vi "Lab_1_Mione_1.vi"() -> ()   [LabVIEW 2018]
panel:
  in  "Current":string
  in  "Temperature":string
  in  "Comment":string
  in  "file path (use dialog)":path
  out "acquiring":bool
  in  "stop acquisition":bool
  in  "Resolution":string(combo)
  in  "Averages":string(combo)
  in  "Enum":T1(ring)=enum."command"
  in  "enter":bool
  in  "stop":bool
  in  "Stop [nm]":dbl
  out "Stop [THz]":dbl
  out "Start [THz]":dbl
  in  "Start [nm]":dbl
  in  "8000/8002":bool
  out "read buffer":string
  in  "Check instruction":string
  out "Initialized":bool
  out "ID number":string
  out "XY Graph":cluster{dbl[], dbl[]}(graph)
  # "Acquisition parameters"
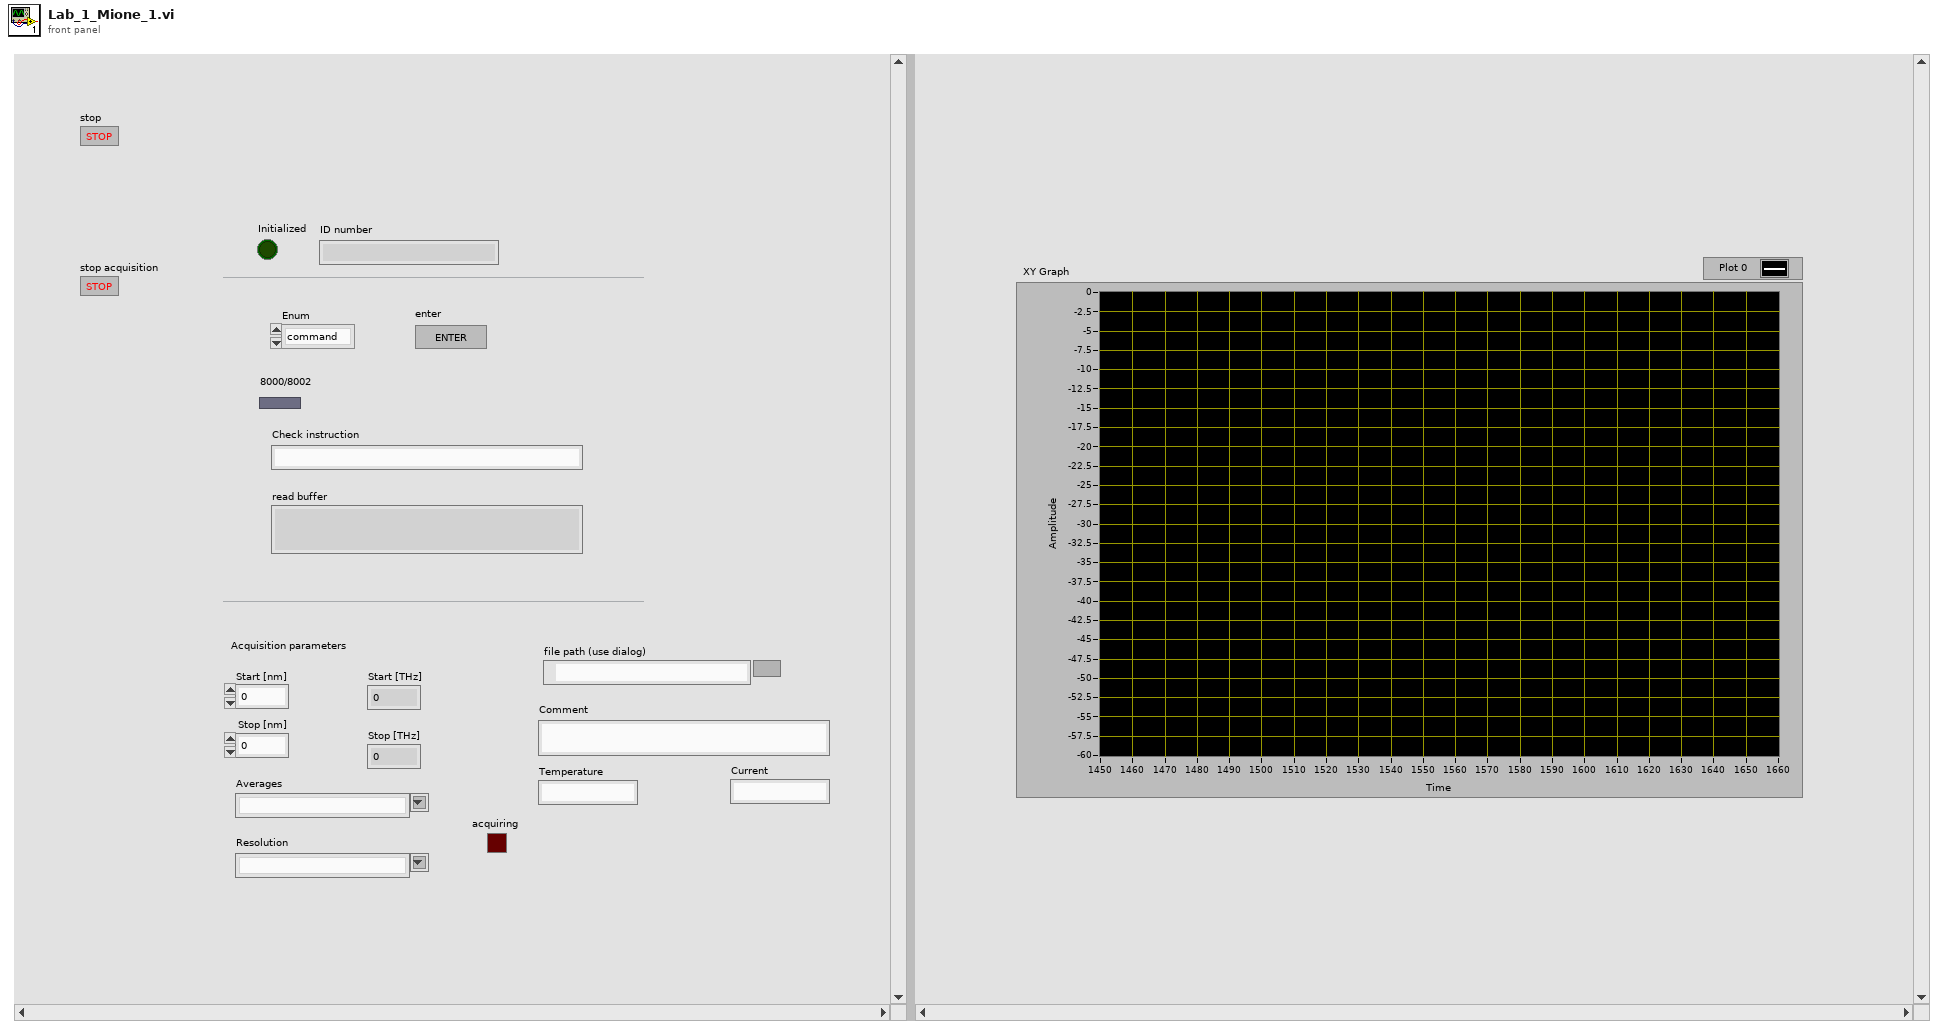
[diagram p1: front panel]
types:
  T1 = enum16{"acquire", "wait", "command", "query", "initialize"}
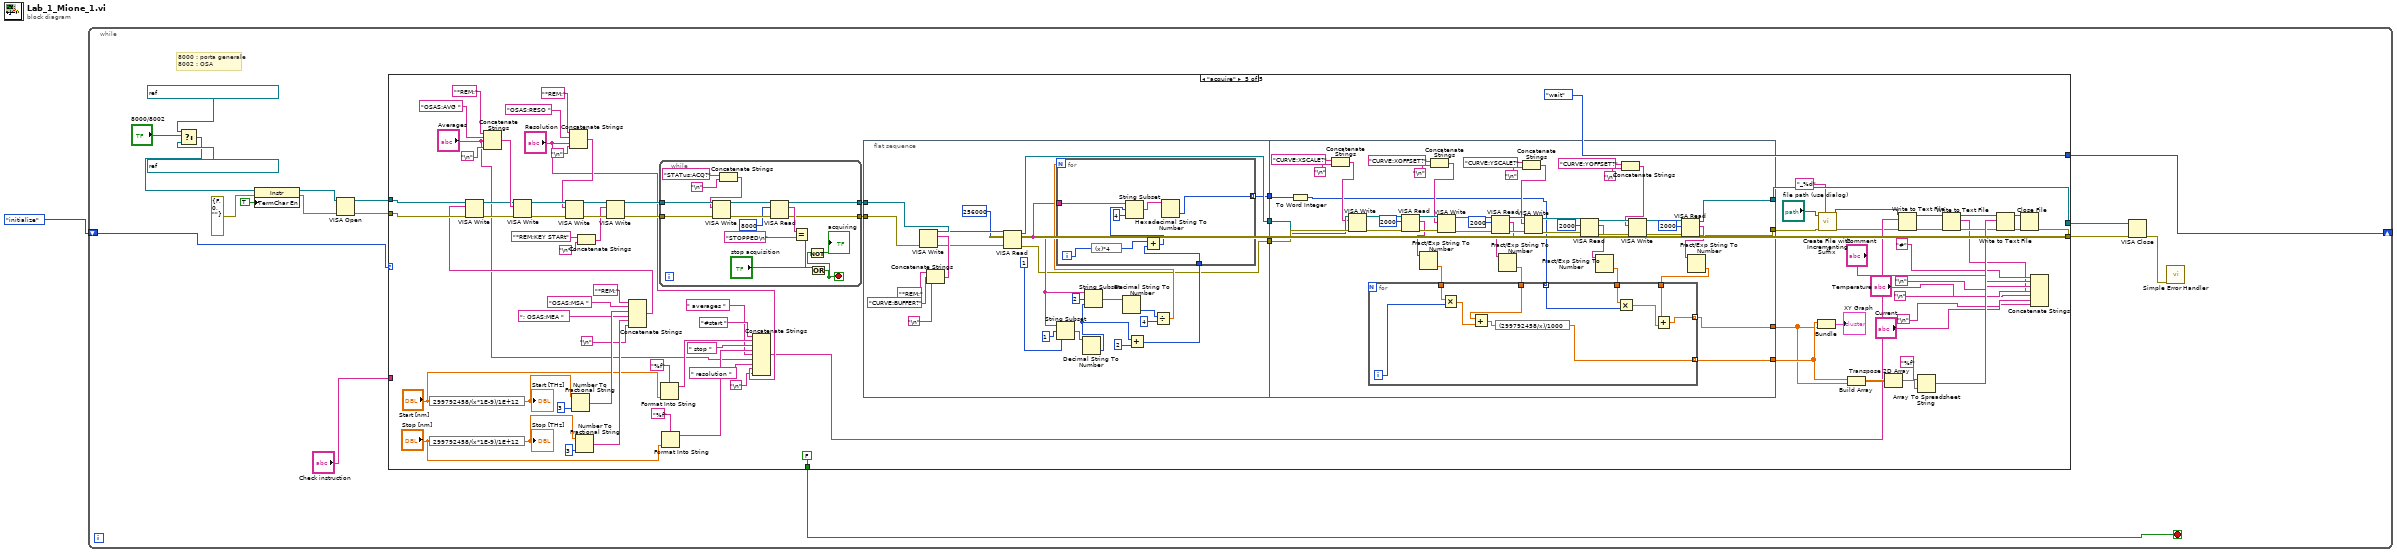
[diagram p0: block diagram]
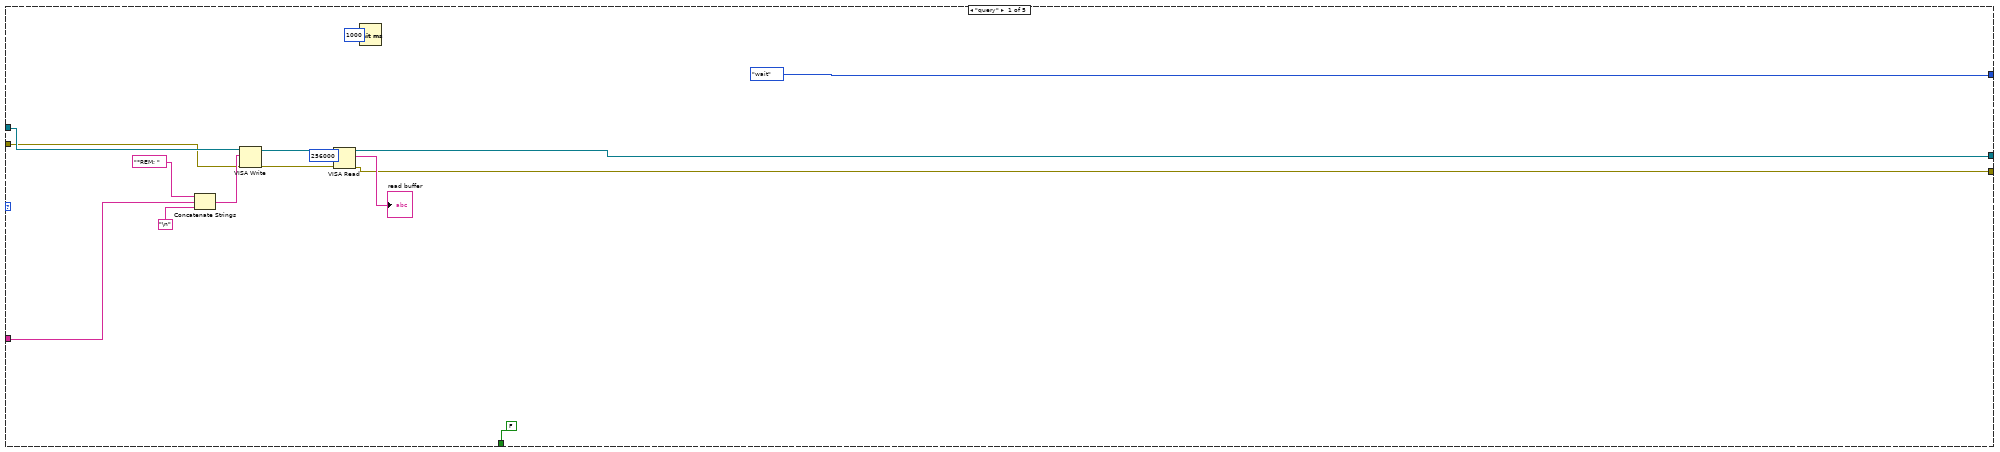
[diagram p2: hidden frame]
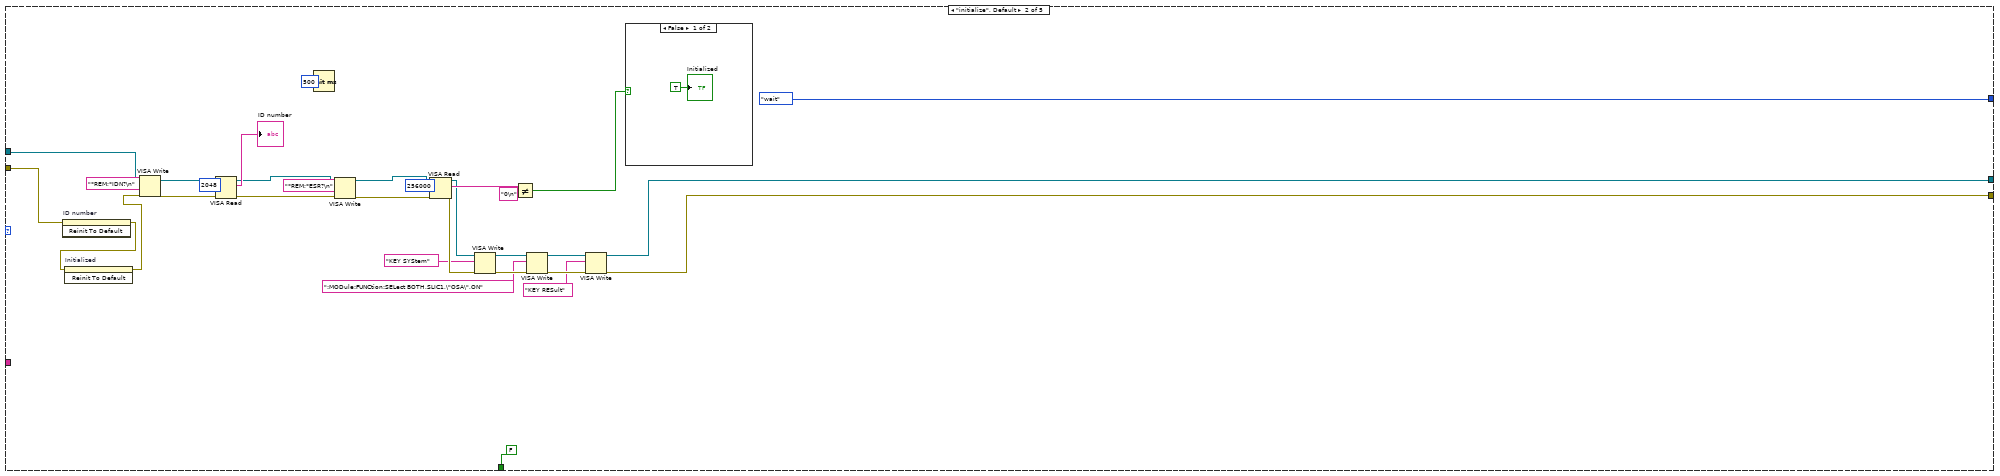
[diagram p3: hidden frame]
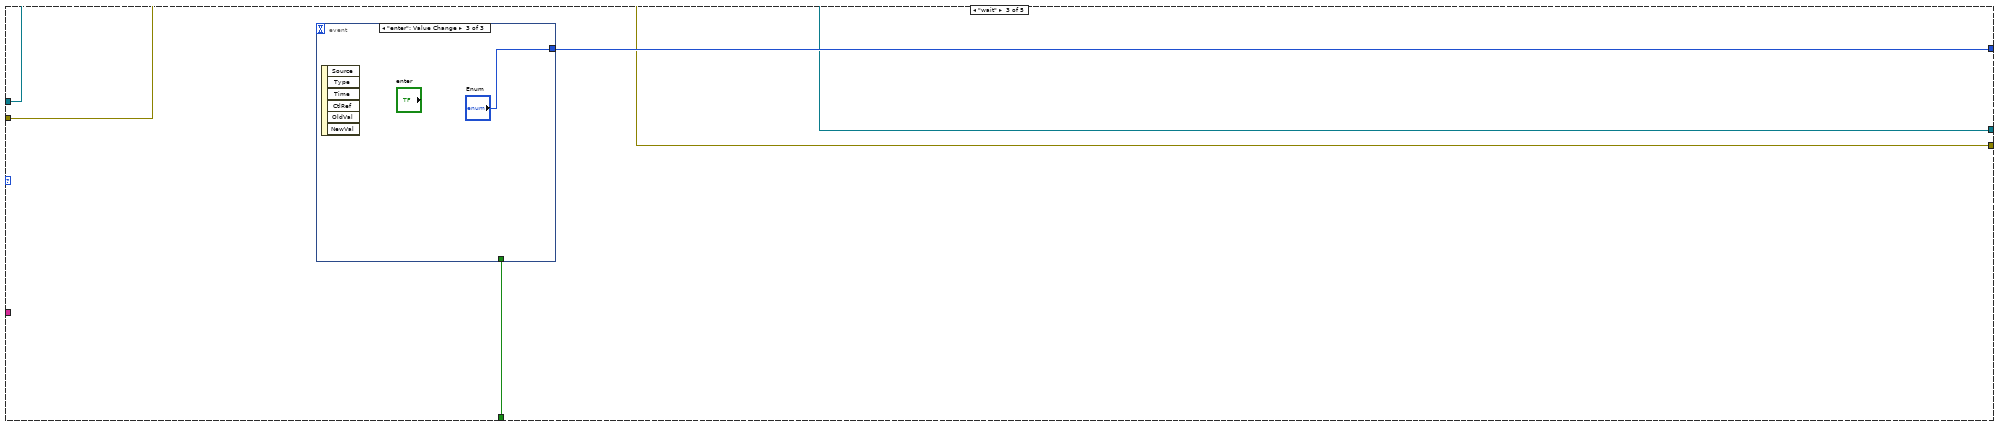
[diagram p5: hidden frame]
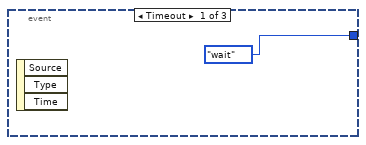
[diagram p6: hidden frame]
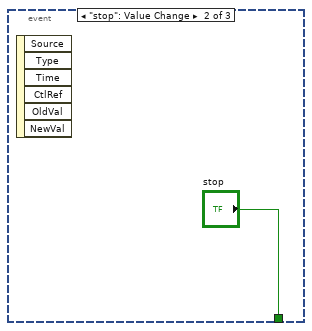
[diagram p7: hidden frame]
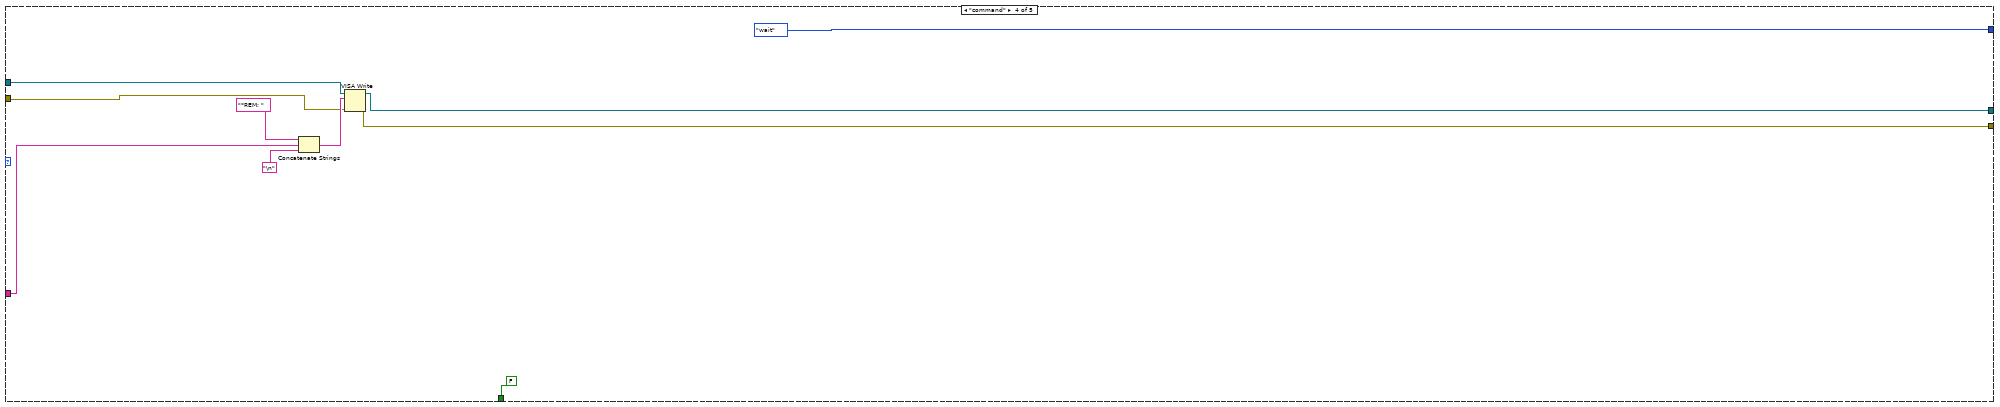
[diagram p8: hidden frame]
diagram:
  n1 = while {
    shift-right: [w9] -> _
    shift-left: T1."initialize" ("Enum") -> [w4]
    stop <- w2 stop-if-true
    # "8000 : porta generale\n8002 : OSA"
    n2 = Select(t=refnum<visa-resource-name> "TCPIP::192.168.121.192::8002::SOCKET" ("VISA resource name"), s="8000/8002", f=refnum<visa-resource-name> "TCPIP::192.168.121.192::8000::SOCKET" ("VISA resource name")) -> (s? t:f=w8:refnum<visa-resource-name>)
    n3 = property class="Instr"(reference=w8, error in=errorcluster {"status"=FALSE, "code"=0, "source"=""} ("error in (no error)"), "TermChar En"=TRUE ("Message Based Settings:Termination Character Enable")) -> (reference out=w6:refnum<visa-resource-name>, error out=w5:errorcluster)
    n4 = VISA Open(error in (no error)=w5, VISA resource name=w6) -> (VISA resource name=w17:refnum<visa-resource-name>, error out=w18:errorcluster)  [unwired: 3 in]
    n5 = case shown="\"acquire\"" w4 {
      tunnel: w18 -> [w30 w47 w67 w79 w152]
      tunnel: w17 -> [w32 w64 w68 w80 w153]
      tunnel: [w25 w35 w68 w78 w120] -> w16
      tunnel: [w24 w34 w67 w77 w116] -> w15
      tunnel: "Check instruction" -> [w21 _ _ w76 _]
      tunnel: [T1."wait" ("Enum") T1."wait" ("Enum") w69 T1."wait" ("Enum") T1."wait" ("Enum")] -> w9
      tunnel: [FALSE ("stop") FALSE ("stop") w70 FALSE ("stop") FALSE ("stop")] -> w2
      frame "query" {
        n6 = Concatenate Strings("*REM; " ("string"), w21, "\n") -> (w31:string)
        n7 = VISA Write(VISA resource name=w32, write buffer=w31, error in (no error)=w30) -> (VISA resource name out=w29:refnum<visa-resource-name>, error out=w28:errorcluster)  [unwired: 1 out]
        n8 = VISA Read(VISA resource name=w29, byte count=u32 256000, error in (no error)=w28) -> (VISA resource name out=w25:refnum<visa-resource-name>, read buffer=→"read buffer":string, error out=w24:errorcluster)  [unwired: 1 out]
        n9 = Wait (ms)(milliseconds to wait=u32 1000) -> ()  [unwired: 1 out]
      }
      frame "initialize", Default {
        n10 = invoke on="ID number" class="Str" method="Reinit To Default"(error in=w47) -> (error out=w46:errorcluster)  [unwired: 2 in, 2 out]
        n11 = invoke on="Initialized" class="Bool (strict)" method="Reinit To Default"(error in=w46) -> (error out=w45:errorcluster)  [unwired: 2 in, 2 out]
        n12 = VISA Write(VISA resource name=w64, write buffer="*REM;*IDN?\n", error in (no error)=w45) -> (VISA resource name out=w63:refnum<visa-resource-name>, error out=w62:errorcluster)  [unwired: 1 out]
        n13 = VISA Read(VISA resource name=w63, byte count=u32 2048, error in (no error)=w62) -> (VISA resource name out=w56:refnum<visa-resource-name>, read buffer=→"ID number":string, error out=w58:errorcluster)  [unwired: 1 out]
        n14 = Wait (ms)(milliseconds to wait=u32 500) -> ()  [unwired: 1 out]
        n15 = VISA Write(VISA resource name=w56, write buffer="*REM;*ESR?\n", error in (no error)=w58) -> (VISA resource name out=w53:refnum<visa-resource-name>, error out=w54:errorcluster)  [unwired: 1 out]
        n16 = VISA Read(VISA resource name=w53, byte count=u32 256000, error in (no error)=w54) -> (VISA resource name out=w44:refnum<visa-resource-name>, read buffer=w50:string, error out=w43:errorcluster)  [unwired: 1 out]
        n17 = VISA Write(VISA resource name=w44, write buffer="KEY SYStem", error in (no error)=w43) -> (VISA resource name out=w41:refnum<visa-resource-name>, error out=w40:errorcluster)  [unwired: 1 out]
        n18 = Not Equal?(x=w50, y="0\n") -> (x != y?=w51:bool)
        n19 = VISA Write(VISA resource name=w41, write buffer=":MODule:FUNCtion:SELect BOTH,SLIC1,\"OSA\",ON", error in (no error)=w40) -> (VISA resource name out=w38:refnum<visa-resource-name>, error out=w37:errorcluster)  [unwired: 1 out]
        n20 = VISA Write(VISA resource name=w38, write buffer="KEY RESult", error in (no error)=w37) -> (VISA resource name out=w35:refnum<visa-resource-name>, error out=w34:errorcluster)  [unwired: 1 out]
        n21 = case shown="False" w51 {
          frame False {
            "Initialized" <- TRUE ("Boolean")
          }
          frame True {
          }
        }
      }
      frame "wait" {
        n22 = event shown="[2] \"enter\": Value Change" {
          selector: _ -> [_ _ _]
          dyn-events: _ -> [_ _ _]
          timeout: _ -> [_ _ _]
          tunnel: [_ "stop" _] -> w70
          tunnel: [T1."wait" ("Enum") _ "Enum"] -> w69
          event Timeout {
            n23 = event-data() -> ()  [unwired: 1 in, 3 out]
          }
          event "stop": Value Change {
            n24 = event-data() -> ()  [unwired: 1 in, 6 out]
          }
          event "enter": Value Change {
            n25 = event-data() -> ()  [unwired: 1 in, 6 out]
          }
        }
      }
      frame "command" {
        n26 = Concatenate Strings("*REM; " ("string"), w76, "\n") -> (w83:string)
        n27 = VISA Write(VISA resource name=w80, write buffer=w83, error in (no error)=w79) -> (VISA resource name out=w78:refnum<visa-resource-name>, error out=w77:errorcluster)  [unwired: 1 out]
      }
      frame "acquire" {
        n28 = expression code="299792458/(x*1E-9)/1E+12"("Start [nm]") -> (w163:dbl)
        "Start [THz]" <- w163
        n29 = expression code="299792458/(x*1E-9)/1E+12"("Stop [nm]") -> (w162:dbl)
        "Stop [THz]" <- w162
        n30 = Concatenate Strings("*REM;" ("string"), "OSAS:AVG " ("string"), "Averages", "\n") -> (w148:string)
        n31 = Concatenate Strings("*REM;" ("string"), "OSAS:RESO " ("string"), "Resolution", "\n") -> (w139:string)
        n32 = Number To Fractional String(number=w163, precision (6)=i16 3) -> (F-format string=w157:string)  [unwired: 2 in]
        n33 = Number To Fractional String(number=w162, precision (6)=i16 3) -> (F-format string=w155:string)  [unwired: 2 in]
        n34 = Concatenate Strings("*REM;KEY STARt", "\n") -> (w134:string)
        n35 = Concatenate Strings("*REM;" ("string"), "OSAS:MSA " ("string"), w157, "; OSAS:MEA " ("string"), w155, "\n") -> (w151:string)
        n36 = VISA Write(VISA resource name=w153, write buffer=w151, error in (no error)=w152) -> (VISA resource name out=w147:refnum<visa-resource-name>, error out=w146:errorcluster)  [unwired: 1 out]
        n37 = VISA Write(VISA resource name=w147, write buffer=w148, error in (no error)=w146) -> (VISA resource name out=w144:refnum<visa-resource-name>, error out=w145:errorcluster)  [unwired: 1 out]
        n38 = VISA Write(VISA resource name=w144, write buffer=w139, error in (no error)=w145) -> (VISA resource name out=w138:refnum<visa-resource-name>, error out=w137:errorcluster)  [unwired: 1 out]
        n39 = VISA Write(VISA resource name=w138, write buffer=w134, error in (no error)=w137) -> (VISA resource name out=w133:refnum<visa-resource-name>, error out=w132:errorcluster)  [unwired: 1 out]
        n40 = while {
          tunnel: w133 -> [w269]
          tunnel: w132 -> [w268]
          tunnel: [w258] -> w130
          tunnel: [w257] -> w131
          stop <- w254 stop-if-true
          n41 = Concatenate Strings("STATus:ACQ?", "\n") -> (w265:string)
          n42 = VISA Write(VISA resource name=w269, write buffer=w265, error in (no error)=w268) -> (VISA resource name out=w264:refnum<visa-resource-name>, error out=w263:errorcluster)  [unwired: 1 out]
          n43 = VISA Read(VISA resource name=w264, byte count=u32 8000, error in (no error)=w263) -> (VISA resource name out=w258:refnum<visa-resource-name>, read buffer=w261:string, error out=w257:errorcluster)  [unwired: 1 out]
          n44 = Equal?(x=w261, y="STOPPED\n") -> (x = y?=w256:bool)
          n45 = Or(x=w256, y="stop acquisition") -> (x .or. y?=w254:bool)
          n46 = Not(x=w254) -> (.not. x?=→"acquiring":bool)
        }
        n47 = Format Into String(format string="%f", "Start [nm]") -> (resulting string=w111:string)  [unwired: 2 in, 1 out]
        n48 = Format Into String(format string="%f", "Stop [nm]") -> (resulting string=w108:string)  [unwired: 2 in, 1 out]
        n49 = Concatenate Strings("#start " ("string"), w111, " stop " ("string"), w108, " averages " ("string"), "Averages", " resolution " ("string"), "Resolution", "\n") -> (w101:string)
        n50 = flat-sequence {
          tunnel: w131 -> [w184]
          tunnel: w130 -> [w183]
          tunnel: [w167] -> w128
          tunnel: [w166] -> w127
          tunnel: [w165] -> w126
          tunnel: w128 -> [w241]
          tunnel: w127 -> [w242]
          tunnel: w126 -> [w198]
          tunnel: [w206] -> w120
          tunnel: [w205] -> w96
          tunnel: [w200] -> w125
          tunnel: [w199] -> w124
          frame #0 {
            n51 = Concatenate Strings("*REM;" ("string"), "CURVE:BUFFER?" ("string"), "\n") -> (w185:string)
            n52 = VISA Write(VISA resource name=w183, write buffer=w185, error in (no error)=w184) -> (VISA resource name out=w182:refnum<visa-resource-name>, error out=w181:errorcluster)  [unwired: 1 out]
            n53 = VISA Read(VISA resource name=w182, byte count=u32 256000, error in (no error)=w181) -> (VISA resource name out=w167:refnum<visa-resource-name>, read buffer=w172:string, error out=w166:errorcluster)  [unwired: 1 out]
            n54 = String Subset(string=w172, offset (0)=1, length (rest)=1 ("length (rest)")) -> (substring=w177:string)
            n55 = Decimal String To Number(string=w177) -> (number=w171:i32)  [unwired: 2 in, 1 out]
            n56 = String Subset(string=w172, offset (0)=2, length (rest)=w171) -> (substring=w176:string)
            n57 = Decimal String To Number(string=w176) -> (number=w175:i32)  [unwired: 2 in, 1 out]
            n58 = Add(x=w171, y=2) -> (x+y=w169:i32)
            n59 = Divide(x=w175, y=4) -> (x/y=w173:dbl)
            n60 = for {
              N: w173 -> [_]
              tunnel: w172 -> [w195]
              tunnel: w169 -> [w192]
              tunnel: [w189] -> w165 mode=indexing
              i -> [w194]
              n61 = expression code="(x)*4"(w194) -> (w191:i32)
              n62 = Add(x=w191, y=w192) -> (x+y=w190:i32)
              n63 = String Subset(string=w195, offset (0)=w190, length (rest)=4 ("length (rest)")) -> (substring=w193:string)
              n64 = Hexadecimal String To Number(string=w193) -> (number=w189:u32)  [unwired: 2 in, 1 out]
            }
          }
          frame #1 {
            n65 = To Word Integer(number=w198) -> (16bit integer=w197:i16[])
            n66 = Concatenate Strings("CURVE:XSCALE?" ("string"), "\n") -> (w220:string)
            n67 = VISA Write(VISA resource name=w241, write buffer=w220, error in (no error)=w242) -> (VISA resource name out=w239:refnum<visa-resource-name>, error out=w240:errorcluster)  [unwired: 1 out]
            n68 = VISA Read(VISA resource name=w239, byte count=u32 2000, error in (no error)=w240) -> (VISA resource name out=w231:refnum<visa-resource-name>, read buffer=w210:string, error out=w232:errorcluster)  [unwired: 1 out]
            n69 = Fract/Exp String To Number(string=w210) -> (number=w204:dbl)  [unwired: 3 in, 1 out]
            n70 = Concatenate Strings("CURVE:XOFFSET?" ("string"), "\n") -> (w213:string)
            n71 = VISA Write(VISA resource name=w231, write buffer=w213, error in (no error)=w232) -> (VISA resource name out=w237:refnum<visa-resource-name>, error out=w238:errorcluster)  [unwired: 1 out]
            n72 = VISA Read(VISA resource name=w237, byte count=u32 2000, error in (no error)=w238) -> (VISA resource name out=w230:refnum<visa-resource-name>, read buffer=w209:string, error out=w229:errorcluster)  [unwired: 1 out]
            n73 = Fract/Exp String To Number(string=w209) -> (number=w203:dbl)  [unwired: 3 in, 1 out]
            n74 = Concatenate Strings("CURVE:YSCALE?" ("string"), "\n") -> (w212:string)
            n75 = VISA Write(VISA resource name=w230, write buffer=w212, error in (no error)=w229) -> (VISA resource name out=w235:refnum<visa-resource-name>, error out=w236:errorcluster)  [unwired: 1 out]
            n76 = VISA Read(VISA resource name=w235, byte count=u32 2000, error in (no error)=w236) -> (VISA resource name out=w228:refnum<visa-resource-name>, read buffer=w208:string, error out=w227:errorcluster)  [unwired: 1 out]
            n77 = Fract/Exp String To Number(string=w208) -> (number=w202:dbl)  [unwired: 3 in, 1 out]
            n78 = Concatenate Strings("CURVE:YOFFSET?" ("string"), "\n") -> (w211:string)
            n79 = VISA Write(VISA resource name=w228, write buffer=w211, error in (no error)=w227) -> (VISA resource name out=w233:refnum<visa-resource-name>, error out=w234:errorcluster)  [unwired: 1 out]
            n80 = VISA Read(VISA resource name=w233, byte count=u32 2000, error in (no error)=w234) -> (VISA resource name out=w206:refnum<visa-resource-name>, read buffer=w207:string, error out=w205:errorcluster)  [unwired: 1 out]
            n81 = Fract/Exp String To Number(string=w207) -> (number=w201:dbl)  [unwired: 3 in, 1 out]
            n82 = for {
              tunnel: w204 -> [w253]
              tunnel: w203 -> [w252]
              tunnel: w202 -> [w249]
              tunnel: w201 -> [w246]
              tunnel: [w245] -> w200 mode=indexing
              tunnel: [w244] -> w199 mode=indexing
              tunnel: w197 -> [w243] mode=indexing
              i -> [w248]
              n83 = Multiply(x=w253, y=w248) -> (x*y=w251:dbl)
              n84 = Add(x=w252, y=w251) -> (x+y=w250:dbl)
              n85 = expression code="(299792458/x)/1000"(w250) -> (w245:dbl)
              n86 = Multiply(x=w249, y=w243) -> (x*y=w247:dbl)
              n87 = Add(x=w246, y=w247) -> (x+y=w244:dbl)
            }
          }
        }
        n88 = Bundle(w125, w124) -> (→"XY Graph":cluster{dbl[], dbl[]})  [unwired: 1 in]
        n89 = call <vilib>:"Create File with Incrementing Suffix.vi"("format string (\" (%d)\")"="_%d" ("format string (\" (%d)\")"), "error in (no error)"=w96, "file path"="file path (use dialog)") -> ("error out"=w93:errorcluster, "refnum out"=w94:refnum<file>)  [unwired: 6 in, 1 out]
        n90 = Build Array(w125, w124) -> (w123:dbl[][])
        n91 = Transpose 2D Array(2D array=w123) -> (transposed array=w119:dbl[][])
        n92 = Write to Text File(file (use dialog)=w94, text=w101, error in=w93) -> (refnum out=w100:refnum<file>, error out=w99:errorcluster)  [unwired: 1 in, 1 out]
        n93 = Array To Spreadsheet String(array=w119, 3:"%f" ("format string")) -> (spreadsheet string=w117:string)  [unwired: 1 in]
        n94 = Concatenate Strings("#", "Comment", "\n", "Temperature", "\n", "Current", "\n") -> (w84:string)
        n95 = Write to Text File(file (use dialog)=w100, text=w84, error in=w99) -> (refnum out=w98:refnum<file>, error out=w97:errorcluster)  [unwired: 1 in, 1 out]
        n96 = Write to Text File(file (use dialog)=w98, text=w117, error in=w97) -> (refnum out=w121:refnum<file>, error out=w122:errorcluster)  [unwired: 1 in, 1 out]
        n97 = Close File(refnum=w121, error in=w122) -> (error out=w116:errorcluster)  [unwired: 1 out]
      }
    }
    n98 = VISA Close(VISA resource name=w16, error in (no error)=w15) -> (error out=w14:errorcluster)
    n99 = call <vilib>:"Simple Error Handler.vi"("error in (no error)"=w14) -> ()  [unwired: 4 in, 5 out]
  }
